vi "MessageQ.vi"(8 "Error In":errorcluster, 9 "State in":string, 10 "QState":T1(ring)=enum."Clear") -> (0 "Error Out":errorcluster, 2 "State Out":string)   [LabVIEW 2017]
doc: "Create States Queue to pass through different cases"
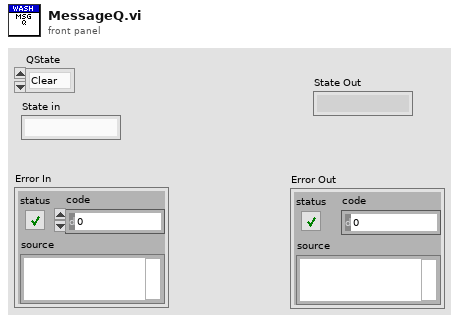
[diagram p1: front panel]
types:
  T1 = enum16{"Create", "Enqueue", "Dequeue", "Enstack", "Flush", "Clear"}
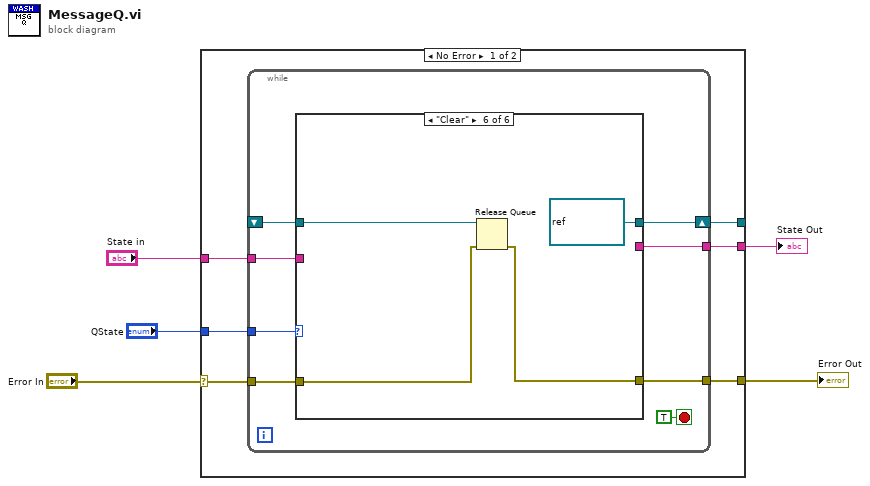
[diagram p0: block diagram]
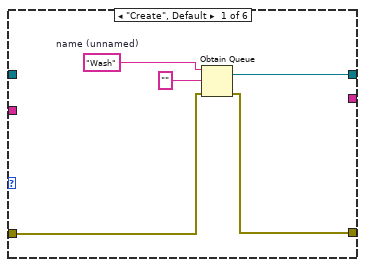
[diagram p2: hidden frame]
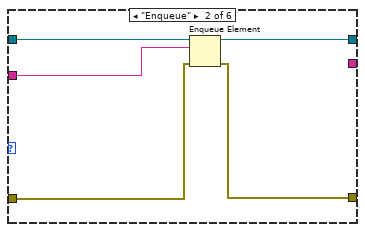
[diagram p3: hidden frame]
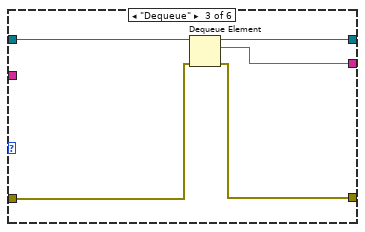
[diagram p4: hidden frame]
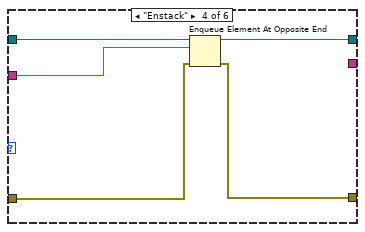
[diagram p5: hidden frame]
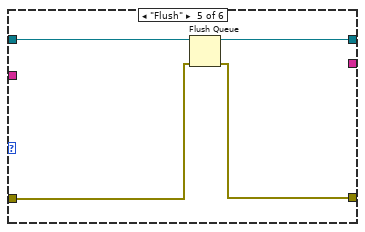
[diagram p6: hidden frame]
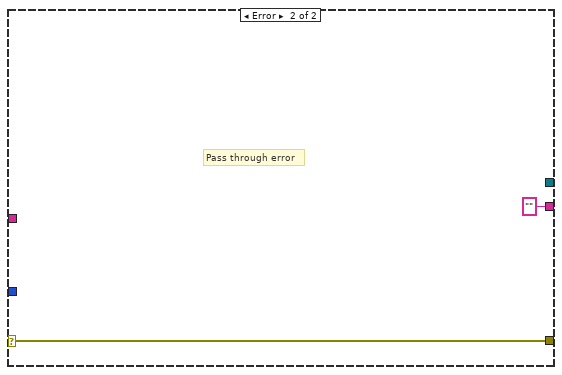
[diagram p7: hidden frame]
diagram:
  n1 = case shown="No Error" "Error In" {
    selector: "Error In" -> [w9 w49]
    tunnel: "QState" -> [w11 _]
    tunnel: [w10 w49] -> w3
    tunnel: [w8 ""] -> w2
    tunnel: "State in" -> [w7 _]
    tunnel: [w6 _] -> _
    frame No Error {
      n2 = while {
        tunnel: w11 -> [w19]
        shift-right: [w18] -> w6
        shift-left: _ -> [w17]
        tunnel: [w15] -> w10
        tunnel: w9 -> [w14]
        tunnel: [w13] -> w8
        tunnel: w7 -> [w12]
        stop <- TRUE stop-if-true
        n3 = case shown="\"Clear\"" w19 {
          tunnel: [w23 w28 w33 w38 w42 refnum<queue> refnum ("queue out")] -> w18
          tunnel: w17 -> [_ w29 w34 w39 w43 w47]
          tunnel: [w20 w26 w31 w36 w40 w45] -> w15
          tunnel: w14 -> [w21 w27 w32 w37 w41 w46]
          tunnel: [_ _ w30 _ _ _] -> w13
          tunnel: w12 -> [_ w25 _ w35 _ _]
          frame "Create", Default {
            w22 = "Wash"  # name (unnamed)
            n4 = Obtain Queue(name (unnamed)=w22, element data type="", error in (no error)=w21) -> (queue out=w23:refnum<queue>, error out=w20:errorcluster)  [unwired: 2 in, 1 out]
          }
          frame "Enqueue" {
            n5 = Enqueue Element(queue=w29, element=w25, error in (no error)=w27) -> (queue out=w28:refnum<queue>, error out=w26:errorcluster)  [unwired: 1 in, 1 out]
          }
          frame "Dequeue" {
            n6 = Dequeue Element(queue=w34, error in (no error)=w32) -> (queue out=w33:refnum<queue>, element=w30:string, error out=w31:errorcluster)  [unwired: 1 in, 1 out]
          }
          frame "Enstack" {
            n7 = Enqueue Element At Opposite End(queue=w39, element=w35, error in (no error)=w37) -> (queue out=w38:refnum<queue>, error out=w36:errorcluster)  [unwired: 1 in, 1 out]
          }
          frame "Flush" {
            n8 = Flush Queue(queue=w43, error in (no error)=w41) -> (queue out=w42:refnum<queue>, error out=w40:errorcluster)  [unwired: 1 out]
          }
          frame "Clear" {
            n9 = Release Queue(queue=w47, error in (no error)=w46) -> (error out=w45:errorcluster)  [unwired: 1 in, 2 out]
          }
        }
      }
    }
    frame Error {
      # "Pass through error"
    }
  }
  "Error Out" <- w3
  "State Out" <- w2
